vi "LiftSystem.vi"(11 "Lift Speed":dbl) -> ()   [LabVIEW 2018]
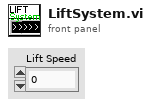
[diagram p1: front panel]
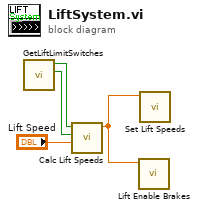
[diagram p0: block diagram]
diagram:
  n1 = call "GetLiftLimitSwitches.vi"() -> ("Lower Limit Switch"=w3:bool, "Upper Limit Switch"=w4:bool)  [unwired: 10 in]
  n2 = call "Calc Lift Speeds.vi"("Lift Speed"="Lift Speed", "Lower Limit Switch"=w3, "Upper Limit Switch"=w4) -> ("Lift Speed"=w2:dbl)  [unwired: 8 in]
  n3 = call "Lift Enable Brakes.vi"("Lift Speed"=w2) -> ()  [unwired: 11 in]
  n4 = call "Set Lift Speeds.vi"("Lift Speed"=w2) -> ()  [unwired: 11 in]
